vi "Get_States_and_Data.vi"(0 "Coffee_Machine_Data":T2={"Backend_Data"={"Level"={"Water_Level"=0.0, "Bean_Level"=0.0, "Milk_Level"=0.0}, "Total_Cups"=0.0}, "Selector"={"Select_Bevarage"=0, "Cup"=FALSE, "Carafe"=FALSE}, "Cup_Unit"=5.0, "Carafe_Unit"=20.0, "Ingreedient_File_PAth"=path "", "Process_Needed"=[], "Indredient_Needed"=[], "Time_Needed"=[], "State_and_Data"={"State"="", "Data"=variant}} {"Backend_Data"."Level"."Milk_Level" scale=0.0..100.0; "Backend_Data"."Level"."Bean_Level" scale=0.0..100.0; "Backend_Data"."Level"."Water_Level" scale=0.0..100.0; "Selector"."Select_Bevarage" scale=0.0..2.0}, 5 "Ingredient_Needed":string[](array[string])) -> (4 "States_and_Data":T1[](array[typedef]))   [LabVIEW 2023]
uses:
  Controls/State_and_Data.ctl
  Controls/Select_Preference.ctl
  Controls/Quantity_Data.ctl
  Controls/Coffee_Machine_Data.ctl
panel:
  # "COFFEE MACHINE"
  # "Backend Control Panel"
  # "Coffee"
  # "Latte"
  # "Hot Water"
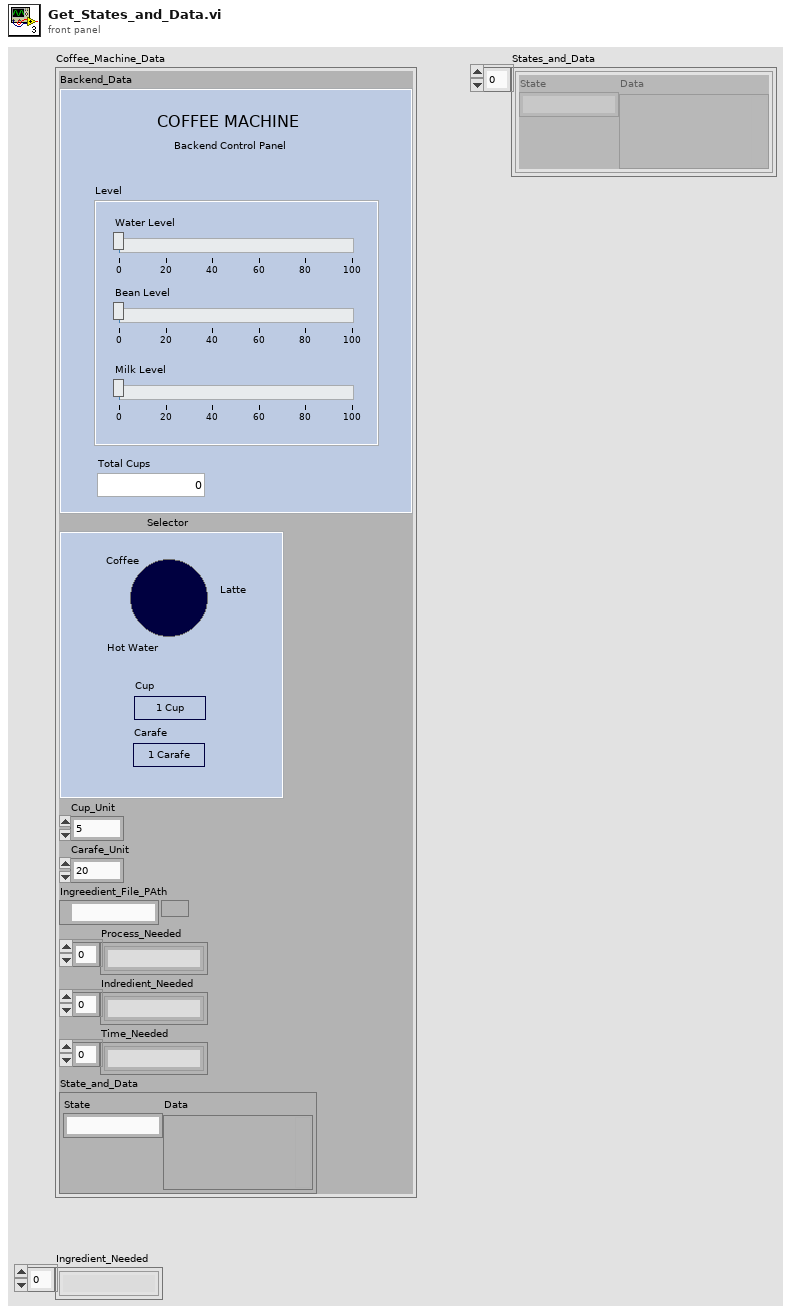
[diagram p1: front panel]
types:
  T1 = typedef "State_and_Data.ctl" = cluster{"State":string, "Data":variant}
  T2 = typedef "Coffee_Machine_Data.ctl" = cluster{"Backend_Data":T3, "Selector":T4, "Cup_Unit":dbl, "Carafe_Unit":dbl, "Ingreedient_File_PAth":path, "Process_Needed":string[], "Indredient_Needed":string[], "Time_Needed":string[], "State_and_Data":T1}
  T3 = typedef "Quantity_Data.ctl" = cluster{"Level":cluster{"Water_Level":dbl, "Bean_Level":dbl, "Milk_Level":dbl}, "Total_Cups":dbl}
  T4 = typedef "Select_Preference.ctl" = cluster{"Select_Bevarage":i32, "Cup":bool, "Carafe":bool}
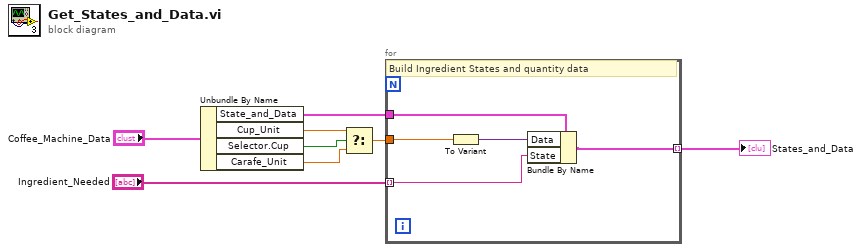
[diagram p0: block diagram]
diagram:
  n1 = Unbundle By Name("Coffee_Machine_Data") -> ("State_and_Data"=w2:T1, "Cup_Unit"=w6:dbl, "Selector.Cup"=w5:bool, "Carafe_Unit"=w7:dbl)
  n2 = Select(t=w6, s=w5, f=w7) -> (s? t:f=w4:dbl)
  n3 = for {
    tunnel: "Ingredient_Needed" -> [w12] mode=indexing
    tunnel: w4 -> [w11]
    tunnel: w2 -> [w13]
    tunnel: [w9] -> w1 mode=indexing
    # "Build Ingredient States and quantity data"
    n4 = To Variant(anything=w11) -> (Variant=w10:variant)
    n5 = Bundle By Name(cluster=w13, "Data"=w10, "State"=w12) -> (w9:T1)
  }
  "States_and_Data" <- w1
